vi "Get UNIX Time.vi"() -> (0 "UNIX seconds":i32)   [LabVIEW 2009]
doc: "This VI returns the number of seconds since 00:00:00, 01Jan1970 UTC, the epoch used on UNIX systems."
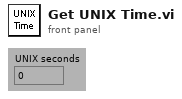
[diagram p1: front panel]
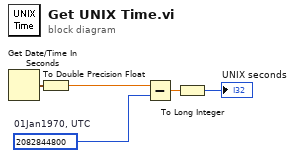
[diagram p0: block diagram]
diagram:
  w4 = 2082844800  # 01Jan1970, UTC
  n1 = Get Date/Time In Seconds() -> (seconds since 1Jan1904=w1:timestamp)
  n2 = To Double Precision Float(number=w1) -> (double precision float=w5:dbl)
  n3 = Subtract(x=w5, y=w4) -> (x-y=w3:dbl)
  n4 = To Long Integer(number=w3) -> (32bit integer=→"UNIX seconds":i32)
